vi "Set Motor Index.vi"(8 "error in (no error)":errorcluster, 10 "Motor Index":u8, 11 "SGDV_Ctrl_Class in":refnum<class "SGDV Motor.lvclass">) -> (0 "error out":errorcluster, 3 "SGDV_Ctrl_Class out":refnum<class "SGDV Motor.lvclass">)   [LabVIEW 2013, in "SGDV_Ctrl_v13_lib.lvlib" / "SGDV Motor.lvclass"]
uses:
  SGDV Motor.lvclass
  SGDV Motor.lvclass/SGDV Motor.ctl
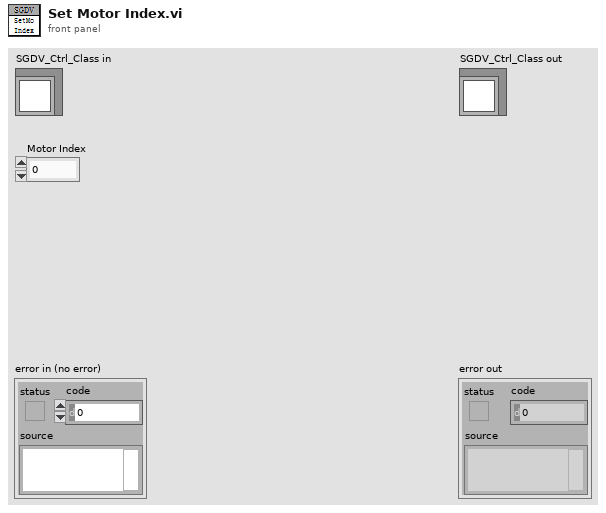
[diagram p1: front panel]
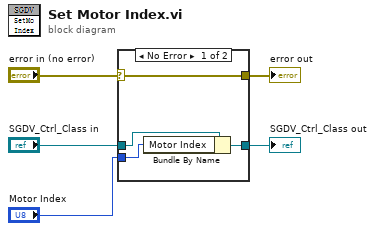
[diagram p0: block diagram]
diagram:
  n1 = case shown="No Error" "error in (no error)" {
    selector: "error in (no error)" -> [w9 w10]
    tunnel: [w9 w10] -> w4
    tunnel: [w7 w11] -> w2
    tunnel: "SGDV_Ctrl_Class in" -> [w8 w11]
    tunnel: "Motor Index" -> [w6 _]
    frame No Error {
      n2 = Bundle By Name(cluster=w8, "Motor Index"=w6) -> (w7:refnum<class "SGDV Motor.lvclass">)
    }
    frame Error {
    }
  }
  "error out" <- w4
  "SGDV_Ctrl_Class out" <- w2
